vi "G#Object_StopExternalCreateProcess.vi"(5 "error in (no error)":errorcluster) -> (15 "stopped?":bool, 19 "error out":errorcluster)   [LabVIEW 2020, in "G#Object.lvclass"]
doc: "Stops then external create process in the background. It is usually stopped when running the garbage collector."
uses:
  <vilib>/addons/_AddQ/G#Object/G#Object.lvclass
  <vilib>/addons/_AddQ/G#Object/utils/G#Object_EventType.ctl
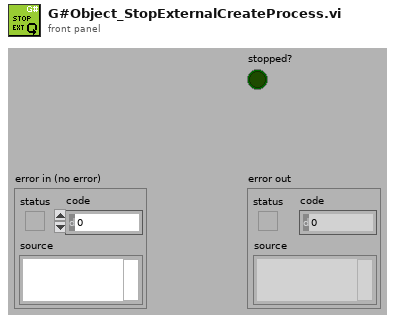
[diagram p1: front panel]
types:
  T1 = enum16{"Initialize", "Register", "Unregister", "Clear"}
  T2 = typedef "G#Object.lvclass/G#Object_EventType.ctl" = enum16{"Created new", "Looked up existing", "Deleted", "Forced delete", "Not deleted", "Garbage collected", "Cleared", "User", "Error", "External create object", "External create class attributes", "Created class attributes", "Run constructor", "Run constructor done", "Run open method", "Run open method done"}
  T3 = enum32{"Bad", "Idle", "Run top level", "Running"}
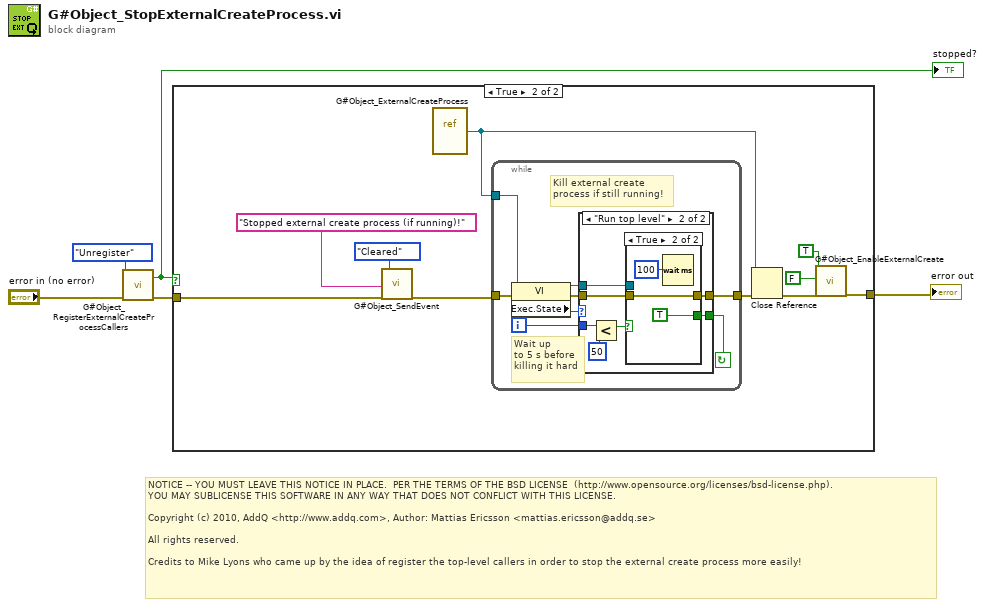
[diagram p0: block diagram]
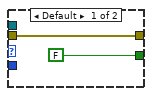
[diagram p3: hidden frame]
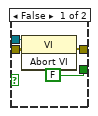
[diagram p4: hidden frame]
diagram:
  # "NOTICE -- YOU MUST LEAVE THIS NOTICE IN PLACE.  PER THE TERMS OF THE BSD LICENSE  (http://www.opensource.org/licenses/bsd-license.php).\nYOU MAY SUBLICENSE THIS SOFTWARE IN ANY WAY THAT DOES NOT CONFLICT WITH THIS LICENSE.\n\nCopyright (c) 2010, AddQ <http://www.addq.com>, Author: Mattias Ericsson <mattias.ericsson@addq.se>\n\nAll rights reserved.\n\nCredits to Mike Lyons who came up by the idea of register the top-level callers in order to stop the external create process more easily!"
  n1 = call <vilib>:"G#Object_RegisterExternalCreateProcessCallers.vi"("Action"=T1."Unregister", "error in (no error)"="error in (no error)") -> ("StopExternalCreate?"=w1:bool, "error out"=w3:errorcluster)  [unwired: 16 in]
  "stopped?" <- w1
  n2 = case shown="True" w1 {
    tunnel: [w6 w7] -> w5
    tunnel: w3 -> [w6 w8]
    frame False {
    }
    frame True {
      n3 = call <vilib>:"G#Object_SendEvent.vi"("comment"="Stopped external create process (if running)!", "error in (no error)"=w8, "G# event type"=G#Object_EventType."Cleared") -> ("error out"=w10:errorcluster)  [unwired: 16 in]
      n4 = vi-ref <vilib>:"G#Object_ExternalCreateProcess.vi"() -> (w12:refnum<vi>)
      n5 = while {
        tunnel: w10 -> [w24]
        tunnel: [w21] -> w13
        tunnel: w12 -> [w19]
        i -> [w17]
        stop <- w18 continue-if-true
        # "Wait up\nto 5 s before\nkilling it hard"
        # "Kill external create\nprocess if still running!"
        n6 = property class="VI"(reference=w19, error in=w24) -> (reference out=w20:refnum<vi>, error out=w22:errorcluster, "Exec.State"=w23:T3)
        n7 = case shown="\"Run top level\"" w23 {
          tunnel: [w26 w29] -> w21
          tunnel: w22 -> [w26 w30]
          tunnel: w20 -> [_ w27]
          tunnel: [FALSE w28] -> w18
          tunnel: w17 -> [_ w33]
          frame Default {
          }
          frame "Run top level" {
            n8 = Less?(x=w33, y=50) -> (x < y?=w31:bool)
            n9 = case shown="True" w31 {
              tunnel: w30 -> [w35 w39]
              tunnel: [w36 w39] -> w29
              tunnel: [FALSE TRUE] -> w28
              tunnel: w27 -> [w34 _]
              frame False {
                n10 = invoke class="VI" method="Abort VI"(reference=w34, error in=w35) -> (error out=w36:errorcluster)  [unwired: 1 in, 2 out]
              }
              frame True {
                n11 = Wait (ms)(milliseconds to wait=u32 100) -> ()  [unwired: 1 out]
              }
            }
          }
        }
      }
      n12 = Close Reference(reference=w12, error in (no error)=w13) -> (error out=w11:errorcluster)
      n13 = call <vilib>:"G#Object_EnableExternalCreate.vi"("set (F)"=TRUE ("set"), "external create enable (F)"=FALSE ("external create enable"), "error in (no error)"=w11) -> ("error out"=w7:errorcluster)  [unwired: 14 in, 2 out]
    }
  }
  "error out" <- w5
